vi "Make Call.vi"(8 "error in (no error)":errorcluster, 11 "Customer With Phone In":refnum<class "Customer With Phone.lvclass">) -> (0 "error out":errorcluster, 3 "Customer With Phone Out":refnum<class "Customer With Phone.lvclass">)   [LabVIEW 2020, in "Customer With Phone.lvclass"]
uses:
  Customer With Phone.lvclass
  <vilib>/Astemes/Triarc Framework/Process/Process.lvclass/Process.ctl
  <vilib>/Astemes/Triarc Framework/Process/Public/Lifecycle/Get Lifecycle State.vi
  <vilib>/Astemes/Triarc Framework/Process/Private/SubVIs/Handle Debug Data.vi
  <vilib>/Utility/error.llb/Clear Errors.vi
  <vilib>/Utility/High Resolution Relative Seconds.vi
  <vilib>/Utility/error.llb/Error Cluster From Error Code.vi
  Customer With Phone.lvclass/Customer With Phone.ctl
  <vilib>/Astemes/Triarc Framework/Process/Process.lvclass
  C:/Git/astemes-triarc-examples/Coffee Shop/Processes/People/Customers/Customer/Customer.lvclass
  C:/Git/astemes-triarc-examples/Coffee Shop/Processes/People/Person/Person.lvclass
  C:/Program Files (x86)/National Instruments/LabVIEW 2020/vi.lib/Astemes/Triarc Framework/View/View.lvclass
  C:/Program Files (x86)/National Instruments/LabVIEW 2020/vi.lib/Astemes/Triarc Framework/Process/Process.lvclass
  C:/Program Files (x86)/National Instruments/LabVIEW 2020/vi.lib/Astemes/Triarc Framework/Base/Base.lvclass
  C:/Program Files (x86)/National Instruments/LabVIEW 2020/vi.lib/Astemes/Triarc Framework/Error Handler Interface/Error Handler Interface.lvclass
  C:/Program Files (x86)/National Instruments/LabVIEW 2020/vi.lib/Astemes/Triarc Framework/Logging/Logging.lvclass
  C:/Git/astemes-triarc-examples/Coffee Shop/Processes/People/Process Job/Job Handler.lvclass
  C:/Program Files (x86)/National Instruments/LabVIEW 2020/vi.lib/Astemes/Triarc Framework/Async Handler/Async Handler.lvclass
  C:/Git/astemes-triarc-examples/Coffee Shop/Processes/People/Customers/Customer With Phone/Customer With Phone.lvclass
  C:/Program Files (x86)/National Instruments/LabVIEW 2020/vi.lib/Astemes/Triarc Framework/Helper Loop/Helper Loop.lvclass
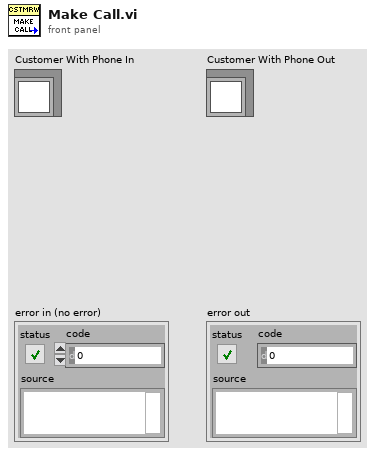
[diagram p1: front panel]
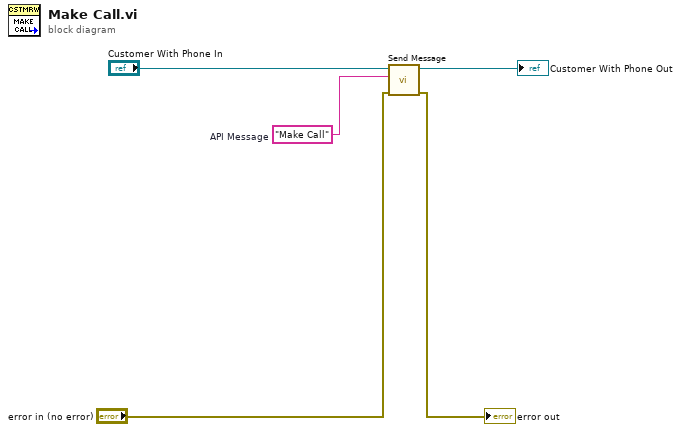
[diagram p0: block diagram]
diagram:
  w2 = "Make Call"  # API Message
  n1 = call <vilib>:"Send Message.vi"("error in (no error)"="error in (no error)", "Message"=w2, "Process In"="Customer With Phone In") -> ("error out"=→"error out":errorcluster, "Process Out"=→"Customer With Phone Out":refnum<class "Customer With Phone.lvclass">)  [unwired: 7 in]
